vi "SPC_start_measurement.vi"(8 "Error In":errorcluster, 10 "Module No":i16 min=0 max=7 step=1, 11 "DLL Path":path) -> (0 "Error Out":errorcluster, 2 "Module No":i16, 3 "DLL Path":path)   [LabVIEW 2023]
doc: "The procedure is used to start the measurement on the SPC module ‘mod_no’.\nBefore a measurement is started by SPC_start_measurement\n- the SPC parameters must be set (SPC_init or SPC_set_parameter(s) ),\n- the SPC memory must be configured ( SPC_configure_memory in normal modes),\n- the measured blocks in SPC memory must be filled (cleared) (SPC_fill_memory),\n- the measurement page must be set (SPC_set_page)\nBecause of hardware differences the procedure action is different for different SPC module types.\nIf the sequencer is not enabled (normal measurement):\n- The repeat and collection timers are started with the specified collect_time\n- The SPC is armed i.e. the photon collection is started.\nIf the sequencer is enabled ('Continuous Flow Mode'):\n If the sequencer is not running:\n - The sequencer is started\n - The SPC is armed for next memory bank. The photon collection is not yet started! This action is not done when sequencer was enabled with ‘enable’ = 2 ( see also SPC_enable_sequencer function ) !\n - SPC is armed for the current memory bank and the photon collection is started.\n If the sequencer is already running:\n - SPC is armed for the current memory bank\n - The memory bank is reversed.\nFor SPC-6x0/13x/830/140/930/15x/160 in FIFO mode:\n- Macro time and FIFO are cleared\n- The SPC is armed i.e. the photon collection is started.\n\ninfo@becker-hickl.com"
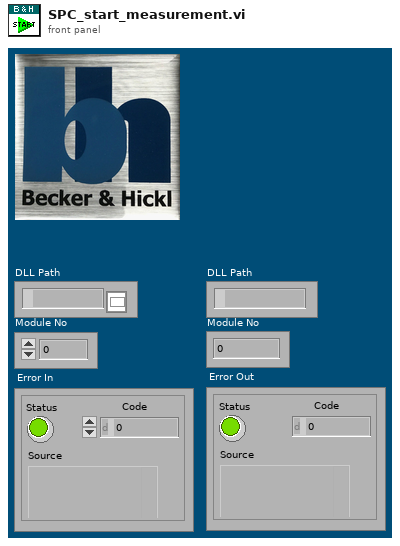
[diagram p1: front panel]
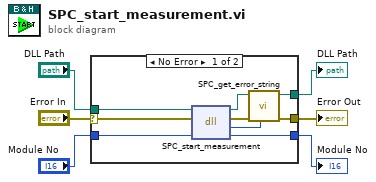
[diagram p0: block diagram]
diagram:
  n1 = case shown="No Error" "Error In" {
    selector: "Error In" -> [w15 w17]
    tunnel: [w9 w17] -> w5
    tunnel: "DLL Path" -> [w14 w18]
    tunnel: [w7 w18] -> w3
    tunnel: "Module No" -> [w13 w16]
    tunnel: [w12 w16] -> w1
    frame No Error {
      n2 = dll-call lib="C:/Program Files (x86)/BH/SPCM/DLL/spcm64.dll" fn="SPC_start_measurement"(path in=w14, error in=w15, "mod_no"=w13) -> (path out=w8:path, error out=w10:errorcluster, "return type"=w11:i16, "mod_no"=w12:i16)  [unwired: 1 in]
      n3 = call "SPC_get_error_string.vi"("ErrorID"=w11, "Error In"=w10, "DLL Path"=w8) -> ("Error Out"=w9:errorcluster, "DLL Path"=w7:path)  [unwired: 6 in, 1 out]
    }
    frame Error {
    }
  }
  "Error Out" <- w5
  "DLL Path" <- w3
  "Module No" <- w1
